vi "Number to Match.vi"() -> ()   [LabVIEW 2019]
panel:
  in  "?":bool
  out "Iteration Count":i32
  in  "Number to Match":i32 min=0 max=100
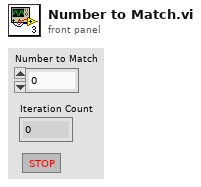
[diagram p1: front panel]
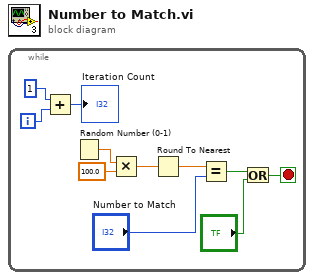
[diagram p0: block diagram]
diagram:
  n1 = while {
    i -> [w10]
    stop <- w1 stop-if-true
    n2 = Add(x=1, y=w10) -> (x+y=→"Iteration Count":i32)
    n3 = Random Number (0-1)() -> (number: 0 to 1=w7:dbl)
    n4 = Multiply(x=w7, y=100.0) -> (x*y=w6:dbl)
    n5 = Round To Nearest(number=w6) -> (nearest integer value=w5:dbl)
    n6 = Equal?(x=w5, y="Number to Match") -> (x = y?=w3:bool)
    n7 = Or(x=w3, y="?") -> (x .or. y?=w1:bool)
  }
